vi "Register Address.vi"(0 "GEA2 Reference In":refnum<k24>, 7 "Address":u8 format="%.0x", 11 "Error In":errorcluster) -> (4 "GEA2 Reference Out":refnum<k24>, 15 "Error Out":errorcluster)   [LabVIEW 2023]
doc: "This VI will register additional source address for the GEA2 bus provided. Messages sent to the additional source address which is registered will then be ACKed by the NewFi device. This is used to minimize additional bus traffic due to extra board responses to messages that would have not been ACKed otherwise."
uses:
  D:/Common/LabVIEW GEA2 Toolkit/source/GEA3 DLL Source/GeaCommunication.dll
  source/GEA3 DLL Source/GeaCommunication.dll
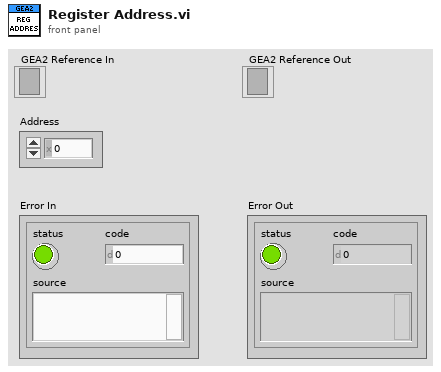
[diagram p1: front panel]
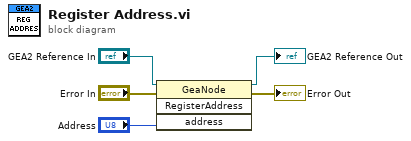
[diagram p0: block diagram]
diagram:
  n1 = invoke class="GeaNode" method="RegisterAddress"(reference="GEA2 Reference In", error in="Error In", "address"="Address") -> (reference out=→"GEA2 Reference Out":refnum<k24>, error out=→"Error Out":errorcluster)  [unwired: 1 in, 2 out]
